vi "FTW-Test-Socket-Stress-SyncServerShutdown.vi"() -> (0 "Test Result":errorcluster)   [LabVIEW 2015]
panel:
  out "Endpoints":string[](array[string])
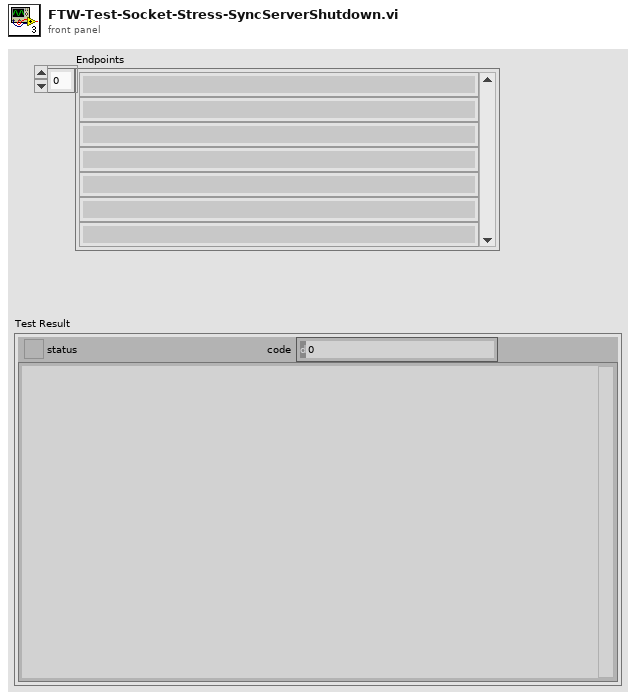
[diagram p1: front panel]
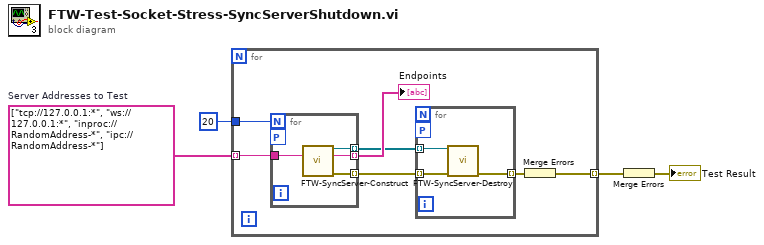
[diagram p0: block diagram]
diagram:
  w4 = string[] ["tcp://127.0.0.1:*", "ws://127.0.0.1:*", "inproc://RandomAddress-*", "ipc://RandomAddress-*"]  # Server Addresses to Test
  n1 = for {
    tunnel: [w5] -> w2 mode=indexing
    tunnel: w4 -> [w7] mode=indexing
    tunnel: 20 -> [w6]
    n2 = for {
      N: w6 -> [_]
      tunnel: [w18] -> w8 mode=indexing
      tunnel: [w17] -> w9 mode=indexing
      tunnel: [w16] -> w11 mode=indexing
      tunnel: w7 -> [w15]
      workers-P: _ -> [_]
      n3 = call "FTW-SyncServer-Construct.vi"("Instance Inbox Address"=w15) -> ("FTW Synchronous Server"=w18:refnum<data-value>, "Resolved Inbox Address"=w17:string, "error out"=w16:errorcluster)  [unwired: 12 in]
    }
    "Endpoints" <- w9
    n4 = for {
      tunnel: w8 -> [w14] mode=indexing
      tunnel: w11 -> [w13] mode=indexing
      tunnel: [w12] -> w10 mode=indexing
      workers-P: _ -> [_]
      n5 = call "FTW-SyncServer-Destroy.vi"("FTW Synchronous Server"=w14, "error in"=w13) -> ("error out"=w12:errorcluster)  [unwired: 13 in]
    }
    n6 = Merge Errors(w10) -> (w5:errorcluster)
  }
  n7 = Merge Errors(w2) -> (→"Test Result":errorcluster)
